vi "PH_PowerUnit_BaseClass.SM State to String.vi"(1 "SM State":T2, 2 "PU":T1) -> (0 "SM State String":string)   [LabVIEW 2014, in "PH_PowerUnit_BaseClass.lvlib"]
uses:
  PH_PowerUnit_BaseClass.lvlib
  PH_PowerUnit_BaseClass.SM States.ctl
  PH_PP_Common/PH_PP_Common.PUs.ctl
  PH_PP_Common/PH_PP_Common.lvlib
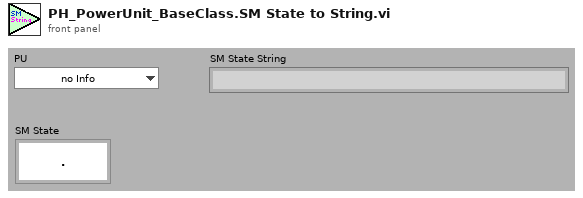
[diagram p1: front panel]
types:
  T1 = typedef "PH_PP_Common.lvlib/PH_PP_Common.PUs.ctl" = enum16{"no Info", "PA-19mm-1", "PA-19mm-2", "PA-45mm-PILC", "PA-45mm-MAIN", "MA-PU-1", "MA-PU-2", "MA-PU-3", "MA-PU-4", "MA-PU-5", "MA-PU-6", "MA-FR", "MA-PILC", "PA-45mm-DP"}
  T2 = typedef "PH_PowerUnit_BaseClass.lvlib/PH_PowerUnit_BaseClass.SM States.ctl" = enum16{".", "Stand by", "Switch PU on", "Configure", "Set Default Voltage", "Set STANDBY", "Set READY", "Wait for Shot Cmd", "Open Dump Rods", "Open Ross Relais", "Close Ross Relais", "Switch PSU on", "Switch PSU off", "Charge", "Switch GD Channel on", "Close Dump Rods", "Rods-TO", "RR-TO", "PSU-TO", "Trigger-TO"}
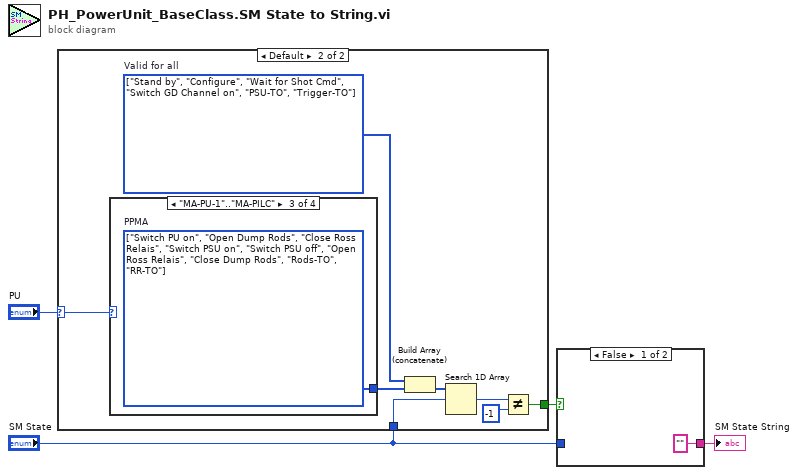
[diagram p0: block diagram]
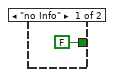
[diagram p2: hidden frame]
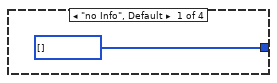
[diagram p3: hidden frame]
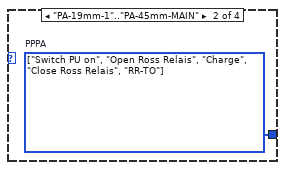
[diagram p4: hidden frame]
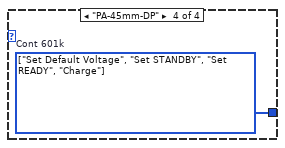
[diagram p5: hidden frame]
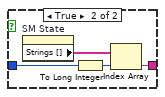
[diagram p6: hidden frame]
diagram:
  n1 = case shown="Default" "PU" {
    selector: "PU" -> [_ w6]
    tunnel: "SM State" -> [_ w8]
    tunnel: [FALSE w7] -> w2
    frame "no Info" {
    }
    frame Default {
      w10 = T2[] [enum."Stand by", enum."Configure", enum."Wait for Shot Cmd", enum."Switch GD Channel on", enum."PSU-TO", enum."Trigger-TO"] items=[".", "Stand by", "Switch PU on", "Configure", "Set Default Voltage", "Set STANDBY", "Set READY", "Wait for Shot Cmd", "Open Dump Rods", "Open Ross Relais", "Close Ross Relais", "Switch PSU on", "Switch PSU off", "Charge", "Switch GD Channel on", "Close Dump Rods", "Rods-TO", "RR-TO", "PSU-TO", "Trigger-TO"]  # Valid for all
      n2 = case shown="\"MA-PU-1\"..\"MA-PILC\"" w6 {
        tunnel: [w14 w15 w16 w17] -> w9
        frame "no Info", Default {
          w14 = T2[] [] items=[".", "Stand by", "Switch PU on", "Configure", "Set Default Voltage", "Set STANDBY", "Set READY", "Wait for Shot Cmd", "Open Dump Rods", "Open Ross Relais", "Close Ross Relais", "Switch PSU on", "Switch PSU off", "Charge", "Switch GD Channel on", "Close Dump Rods", "Rods-TO", "RR-TO", "PSU-TO", "Trigger-TO"] ("Cont 601k")
        }
        frame "PA-19mm-1".."PA-45mm-MAIN" {
          w15 = T2[] [enum."Switch PU on", enum."Open Ross Relais", enum."Charge", enum."Close Ross Relais", enum."RR-TO"] items=[".", "Stand by", "Switch PU on", "Configure", "Set Default Voltage", "Set STANDBY", "Set READY", "Wait for Shot Cmd", "Open Dump Rods", "Open Ross Relais", "Close Ross Relais", "Switch PSU on", "Switch PSU off", "Charge", "Switch GD Channel on", "Close Dump Rods", "Rods-TO", "RR-TO", "PSU-TO", "Trigger-TO"]  # PPPA
        }
        frame "MA-PU-1".."MA-PILC" {
          w16 = T2[] [enum."Switch PU on", enum."Open Dump Rods", enum."Close Ross Relais", enum."Switch PSU on", enum."Switch PSU off", enum."Open Ross Relais", enum."Close Dump Rods", enum."Rods-TO", enum."RR-TO"] items=[".", "Stand by", "Switch PU on", "Configure", "Set Default Voltage", "Set STANDBY", "Set READY", "Wait for Shot Cmd", "Open Dump Rods", "Open Ross Relais", "Close Ross Relais", "Switch PSU on", "Switch PSU off", "Charge", "Switch GD Channel on", "Close Dump Rods", "Rods-TO", "RR-TO", "PSU-TO", "Trigger-TO"]  # PPMA
        }
        frame "PA-45mm-DP" {
          w17 = T2[] [enum."Set Default Voltage", enum."Set STANDBY", enum."Set READY", enum."Charge"] items=[".", "Stand by", "Switch PU on", "Configure", "Set Default Voltage", "Set STANDBY", "Set READY", "Wait for Shot Cmd", "Open Dump Rods", "Open Ross Relais", "Close Ross Relais", "Switch PSU on", "Switch PSU off", "Charge", "Switch GD Channel on", "Close Dump Rods", "Rods-TO", "RR-TO", "PSU-TO", "Trigger-TO"]  # Cont 601k
        }
      }
      n3 = Build Array (concatenate)(w10, w9) -> (w13:T2[])
      n4 = Search 1D Array(1D array=w13, element=w8) -> (index of element=w11:i32)  [unwired: 1 in]
      n5 = Not Equal?(x=w11, y=-1) -> (x != y?=w7:bool)
    }
  }
  n6 = case shown="False" w2 {
    tunnel: ["" w20] -> w4
    tunnel: "SM State" -> [_ w21]
    frame False {
    }
    frame True {
      n7 = property on="SM State" class="Enum (strict)"() -> ("Strings []"=w19:string[])  [unwired: 2 in, 2 out]
      n8 = To Long Integer(number=w21) -> (32bit integer=w22:i32)
      n9 = Index Array(array=w19, index=w22) -> (element=w20:string)
    }
  }
  "SM State String" <- w4
